vi "API_DB.UpdateReticleLocationStatus.vi"(5 "Table":string, 6 "Timeout (ms)":u32, 7 "Wait (F)":bool, 8 "error in (no error)":errorcluster, 9 "InventoryRecord.ReticleID":string, 10 "InventoryRecord.LocationStatus":T1, 11 "Database in":refnum<class "Database.lvclass">) -> (0 "error out":errorcluster, 2 "Slot":string, 3 "Database out":refnum<class "Database.lvclass">)   [LabVIEW 2020, in "Database.lvclass"]
doc: "Developed by Kevin Thompson\nkevin@thompsonengineering.net\n\nCopyright 2018\nThompson Engineering, LLC"
uses:
  Database.lvclass
  DataTypes/LocationStatus--Enum.ctl
  DataTypes/AsynCmd_Temp01--enum.ctl
  DataTypes/GenericQuery--Cluster.ctl
  DataTypes/SQLQuery--Enum.ctl
  DataTypes/InventoryRecord--Cluster.ctl
  DataTypes/Stocker--Enum.ctl
  DataTypes/Module--Cluster.ctl
  Database.lvclass/Database.ctl
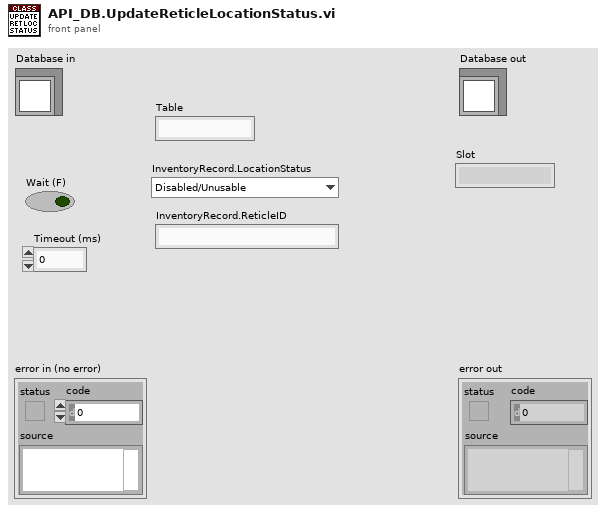
[diagram p1: front panel]
types:
  T1 = typedef "LocationStatus--Enum.ctl" = enum16{"Disabled/Unusable", "Full", "Empty"}
  T2 = typedef "SQLQuery--Enum.ctl" = enum16{"GetInventoryRecordFromDB", "GetReticleInfoFromDB", "GetLocationStatusFromDB", "UpdateInventoryRecord", "UpdateLocationStatus", "UpdateReticleLocationStatus", "AddReticleInDB", "RemoveReticleAtLocation", "RemoveReticleUsingReticleID", "GetLocationForReticleID", "GetAllLocations", "GetAllEmptyLocations", "GetAllLocationsInStocker", "GetAllFullLocations", "GetAllFullLocationsInStocker", "GetAllDisabledLocations", "GetAllDisabledLocationsInStocker", "FindFirstSlot"}
  T3 = typedef "GenericQuery--Cluster.ctl" = cluster{"Query":T2, "Table":string, "InventoryRecord":T4}
  T4 = typedef "InventoryRecord--Cluster.ctl" = cluster{"ReticleID":string, "Stocker":T5, "Location":T6, "LocationStatus":T1, "EquipmentID":string, "LocationID":string}
  T5 = typedef "Stocker--Enum.ctl" = u16
  T6 = typedef "Module--Cluster.ctl" = cluster{"Module":u16, "Row":u16, "Column":u16}
  T7 = typedef "Database.lvclass/AsynCmd_Temp01--enum.ctl" = enum16{"DB.DeleteRecord", "DB.UpdateRecord", "DB.InsertRecord", "DB.SelectRecord", "DB.ExecuteSQLCommand", "DB.FindFirstSlot", "DB.GenericSQLQuery"}
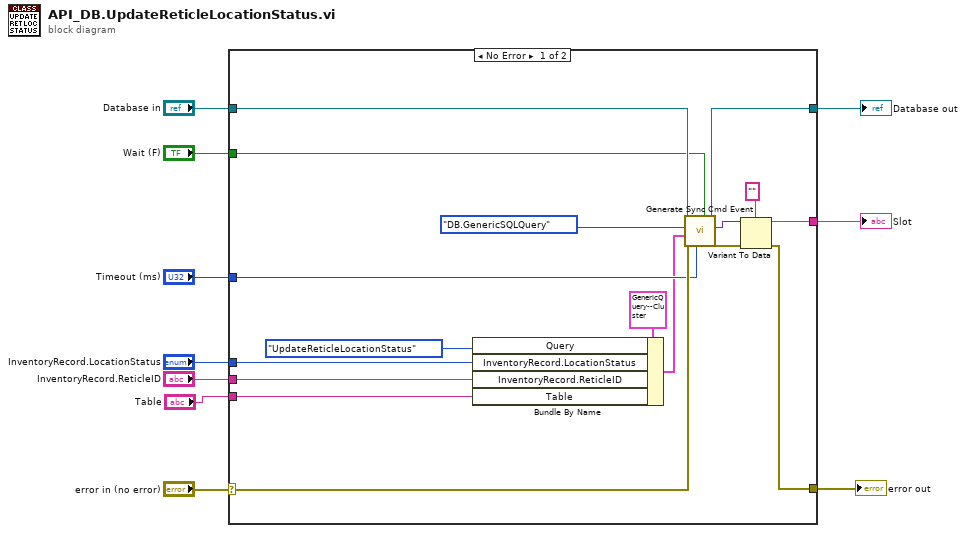
[diagram p0: block diagram]
diagram:
  n1 = case shown="No Error" "error in (no error)" {
    selector: "error in (no error)" -> [w25 w29]
    tunnel: [w20 w29] -> w9
    tunnel: [w26 w28] -> w7
    tunnel: "Database in" -> [w27 w28]
    tunnel: [w22 _] -> w4
    tunnel: "Wait (F)" -> [w19 _]
    tunnel: "Timeout (ms)" -> [w18 _]
    tunnel: "InventoryRecord.ReticleID" -> [w13 _]
    tunnel: "InventoryRecord.LocationStatus" -> [w12 _]
    tunnel: "Table" -> [w11 _]
    frame No Error {
      n2 = Bundle By Name(cluster=T3 {"Query"=enum."GetInventoryRecordFromDB", "Table"="", "InventoryRecord"={"ReticleID"="", "Stocker"=0, "Location"={"Module"=0, "Row"=0, "Column"=0}, "LocationStatus"=enum."Disabled/Unusable", "EquipmentID"="", "LocationID"=""}}, "Query"=SQLQuery--Enum."UpdateReticleLocationStatus", "InventoryRecord.LocationStatus"=w12, "InventoryRecord.ReticleID"=w13, "Table"=w11) -> (w14:T3)
      n3 = call "Generate Sync Cmd Event.vi"("Wait (F)"=w19, "Timeout (ms)"=w18, "error in (no error)"=w25, "vData"=w14, "AsyncCmd"=AsynCmd_Temp01--enum."DB.GenericSQLQuery", "Database in"=w27) -> ("error out"=w21:errorcluster, "Return Value"=w23:variant, "Database out"=w26:refnum<class "Database.lvclass">)  [unwired: 3 in]
      n4 = Variant To Data(error in=w21, type="", Variant=w23) -> (data=w22:string, error out=w20:errorcluster)
    }
    frame Error {
    }
  }
  "error out" <- w9
  "Database out" <- w7
  "Slot" <- w4
